vi "FGV PNS Istwerte.vi"(11 "Störungen 193-256":u64, 12 "Aktionen":T3, 13 "Cluster":cluster{"UsrVal":u16[], "Alarm":T1, "Regler":T2}, 14 "Speicher Freigabe":bool) -> (4 "Regler":T2, 6 "Alarme":T1[](array[typedef]), 8 "UsrVal":u16[](array[numeric]), 15 "Störungen 193-256 2":u64)   [LabVIEW 2020, in "PNS.lvlib"]
uses:
  PNS.lvlib
  Aktionen FGV Istwerte.ctl
  ObjektKlassen/Steuerung PNS/Alarme.ctl
  ObjektKlassen/Steuerung PNS/Regler.ctl
  ObjektKlassen/Steuerung PNS/Steuerung PNS.lvclass
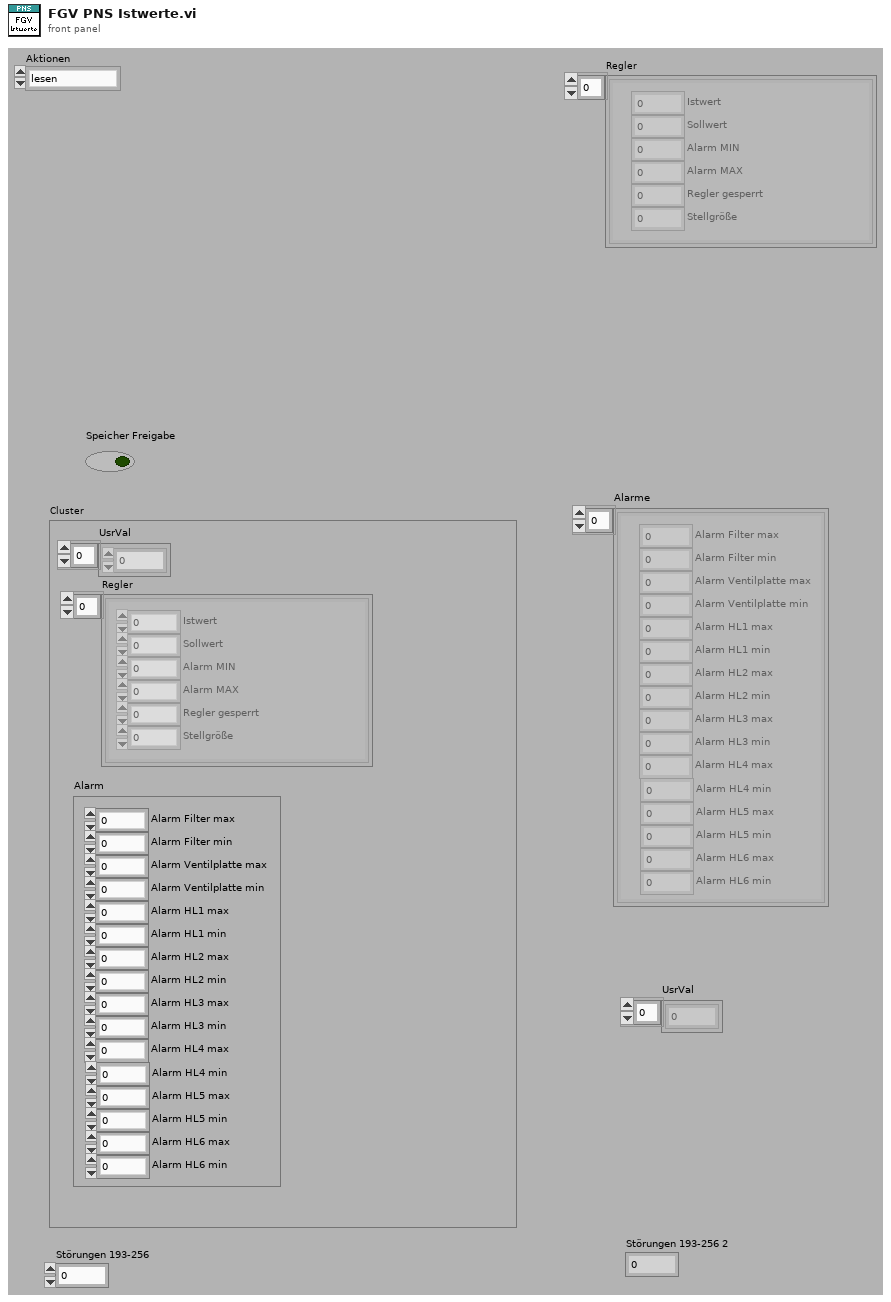
[diagram p1: front panel]
types:
  T1 = typedef "Steuerung PNS.lvclass/Alarme.ctl" = cluster{"Alarm Filter max":u16, "Alarm Filter min":u16, "Alarm Ventilplatte max":u16, "Alarm Ventilplatte min":u16, "Alarm HL1 max":u16, "Alarm HL1 min":u16, "Alarm HL2 max":u16, "Alarm HL2 min":u16, "Alarm HL3 max":u16, "Alarm HL3 min":u16, "Alarm HL4 max":u16, "Alarm HL4 min":u16, "Alarm HL5 max":u16, "Alarm HL5 min":u16, "Alarm HL6 max":u16, "Alarm HL6 min":u16}
  T2 = typedef "Steuerung PNS.lvclass/Regler.ctl" = cluster{"Istwert":i16, "Sollwert":i16, "Alarm MIN":i16, "Alarm MAX":i16, "Regler sperren":i16, "Analog Ausgang":i16}[]
  T3 = typedef "PNS.lvlib/Aktionen FGV Istwerte.ctl" = enum16{"lesen", "initialisieren", "schreiben", "Störungen"}
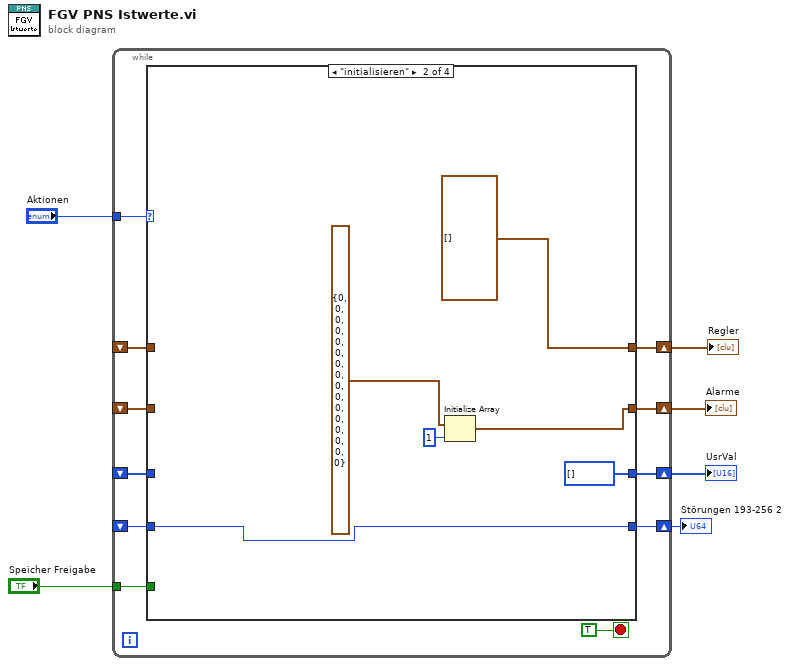
[diagram p0: block diagram]
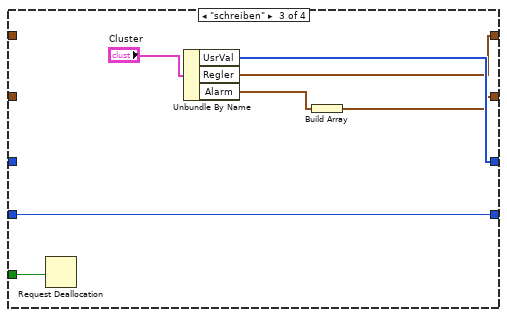
[diagram p3: hidden frame]
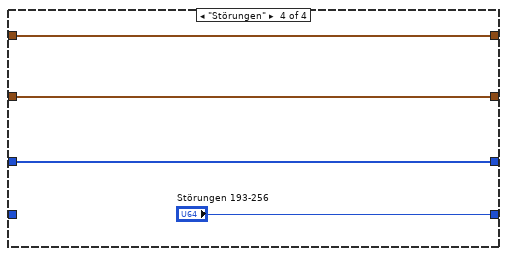
[diagram p4: hidden frame]
diagram:
  n1 = while {
    tunnel: "Aktionen" -> [w17]
    shift-right: [w11] -> w2
    shift-left: _ -> [w12]
    shift-right: [w9] -> w5
    shift-left: _ -> [w13]
    shift-right: [w15] -> w4
    shift-left: _ -> [w14]
    tunnel: "Speicher Freigabe" -> [w10]
    shift-right: [w8] -> w1
    shift-left: _ -> [w7]
    stop <- TRUE stop-if-true
    n2 = case shown="\"initialisieren\"" w17 {
      tunnel: [w19 u16[] [] ("Eingangs Array") w33 w37] -> w15
      tunnel: w14 -> [w19 _ _ w37]
      tunnel: w13 -> [w20 _ _ w36]
      tunnel: w12 -> [w21 _ _ w35]
      tunnel: [w21 T2 [] ("Regler") w32 w35] -> w11
      tunnel: [w20 w25 w30 w36] -> w9
      tunnel: w10 -> [_ _ w28 _]
      tunnel: [w18 w22 w29 "Störungen 193-256"] -> w8
      tunnel: w7 -> [w18 w22 w29 _]
      frame "lesen", Default {
      }
      frame "initialisieren" {
        n3 = Initialize Array(T1 {"Alarm Filter max"=0, "Alarm Filter min"=0, "Alarm Ventilplatte max"=0, "Alarm Ventilplatte min"=0, "Alarm HL1 max"=0, "Alarm HL1 min"=0, "Alarm HL2 max"=0, "Alarm HL2 min"=0, "Alarm HL3 max"=0, "Alarm HL3 min"=0, "Alarm HL4 max"=0, "Alarm HL4 min"=0, "Alarm HL5 max"=0, "Alarm HL5 min"=0, "Alarm HL6 max"=0, "Alarm HL6 min"=0} ("Alarm"), 1 ("Dimension")) -> (w25:T1[])
      }
      frame "schreiben" {
        n4 = Request Deallocation(w28) -> ()
        n5 = Unbundle By Name("Cluster") -> ("UsrVal"=w33:u16[], "Regler"=w32:T2, "Alarm"=w31:T1)
        n6 = Build Array(w31) -> (w30:T1[])
      }
      frame "Störungen" {
      }
    }
  }
  "Alarme" <- w5
  "UsrVal" <- w4
  "Regler" <- w2
  "Störungen 193-256 2" <- w1
